vi "HallR_to_B.vi"(10 "Measured R(Ohm)":dbl, 11 "Calibration Curve Data":dbl[][](array[numeric])) -> (3 "Interpolated B value":dbl)   [LabVIEW 2015]
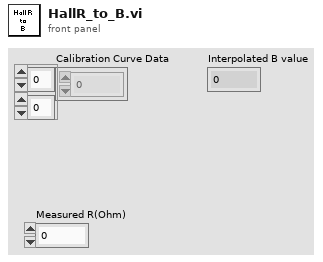
[diagram p1: front panel]
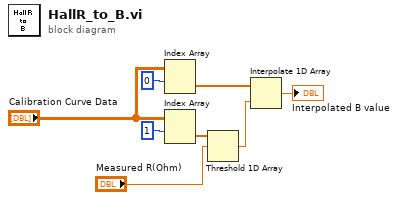
[diagram p0: block diagram]
diagram:
  n1 = Index Array(array="Calibration Curve Data", index (row)=0) -> (element=w6:dbl[])  [unwired: 1 in]
  n2 = Index Array(array="Calibration Curve Data", index (row)=1) -> (element=w8:dbl[])  [unwired: 1 in]
  n3 = Threshold 1D Array(2:"Measured R(Ohm)", 3:w8) -> (0:w7:dbl)  [unwired: 1 in]
  n4 = Interpolate 1D Array(1:w7, 2:w6) -> (0:→"Interpolated B value":dbl)
